vi "Get Array as Variant.vi"(8 "error in (no error)":errorcluster, 10 "Variant (Data Type)":variant, 11 "JSON Value in":refnum<class "JSON Value.lvclass">) -> (0 "error out":errorcluster, 2 "Default VData":variant)   [LabVIEW 2011, in "Variant JSON.lvlib"]
uses:
  Variant JSON.lvlib
  JSON Value/JSON Value.lvclass
  JSON Scalar/Get as I32.vi
  JSON Scalar/Get as I64.vi
  JSON Scalar/Get as U32.vi
  JSON Scalar/Get as SGL.vi
  JSON Scalar/Get as DBL.vi
  JSON Scalar/Get as EXT.vi
  JSON Scalar/Get as Boolean.vi
  JSON Scalar/Get as Text.vi
  JSON Scalar/Get as Path.vi
  JSON Value/Get as Waveform.vi
  JSON Scalar/Get as Timestamp.vi
  JSON Scalar/Get as U64.vi
  <vilib>/Utility/VariantDataType/VariantType.lvlib
  Get Polymorphic/JSON GetSet.lvlib
  JSON Scalar/JSON Scalar.lvclass
  JSON Object/JSON Object.lvclass
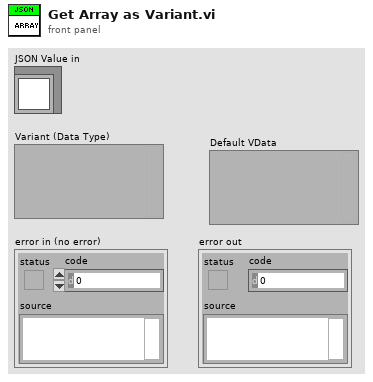
[diagram p1: front panel]
types:
  T1 = typedef "VariantType.lvlib/Type.ctl" = enum8{"Invalid Type", "Void", "I8", "I16", "I32", "I64", "U8", "U16", "U32", "U64", "Single Float", "Double Float", "Extended Float", "Single Complex", "Double Complex", "Extended Complex", "Enum U8", "Enum U16", "Enum U32", "Enum U64", "Single Float With Unit", "Double Float With Unit", "Extended Float With Unit", "Single Complex with Unit", "Double Complex with Unit", "Extended Complex with Unit", "Boolean", "String", "Path", "Picture", "Tag", "Array", "Cluster", "Variant", "LV Variant", "Waveform", "Timestamp", "Digital Waveform", "Digital Data", "ExpressData", "Refnum", "External Data", "VI", "Poly VI", "LabVIEW Class Instance", "Fixed Point"}
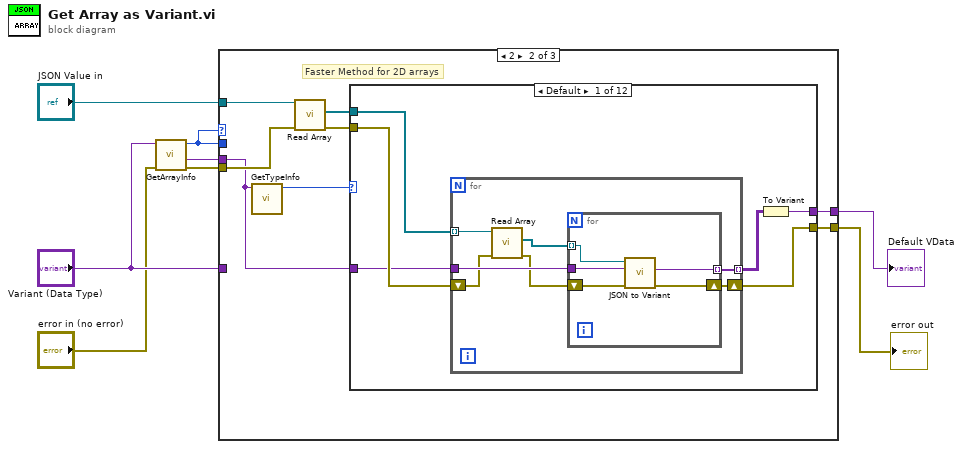
[diagram p0: block diagram]
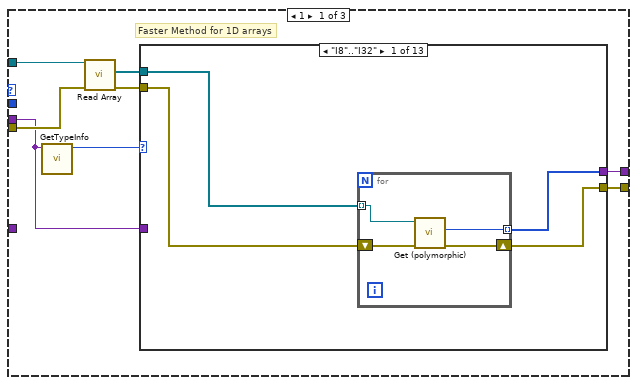
[diagram p2: hidden frame]
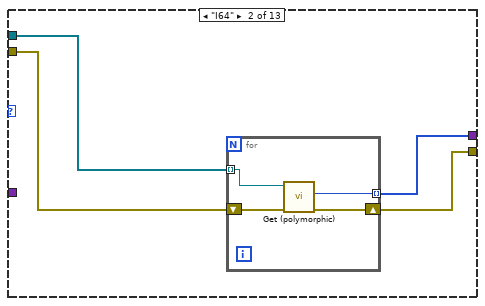
[diagram p3: hidden frame]
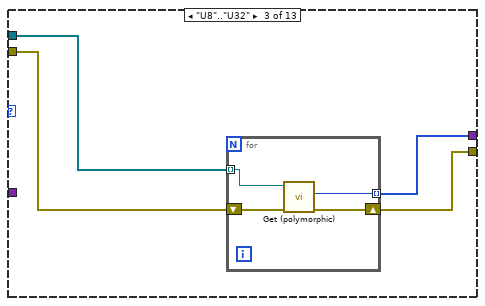
[diagram p4: hidden frame]
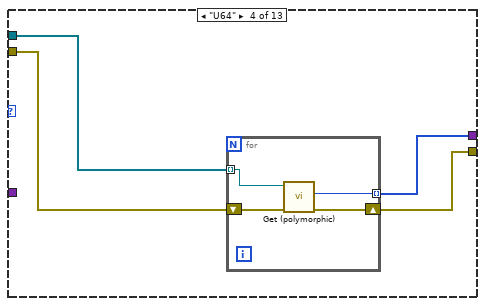
[diagram p5: hidden frame]
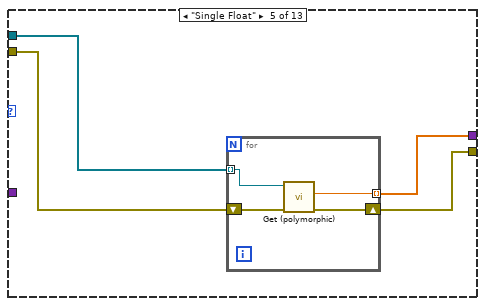
[diagram p6: hidden frame]
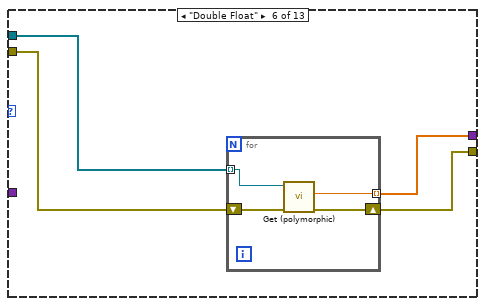
[diagram p7: hidden frame]
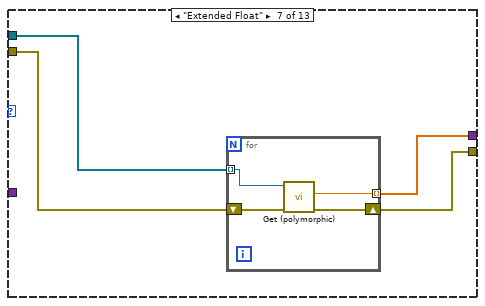
[diagram p8: hidden frame]
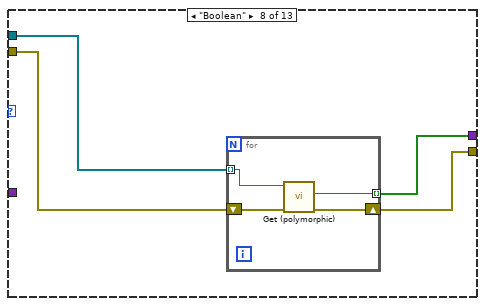
[diagram p9: hidden frame]
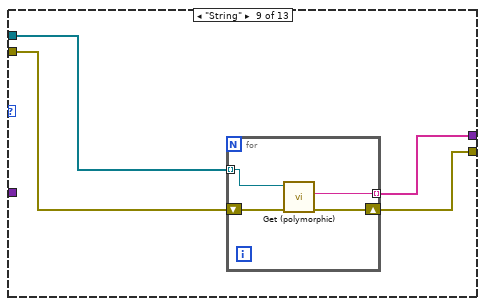
[diagram p10: hidden frame]
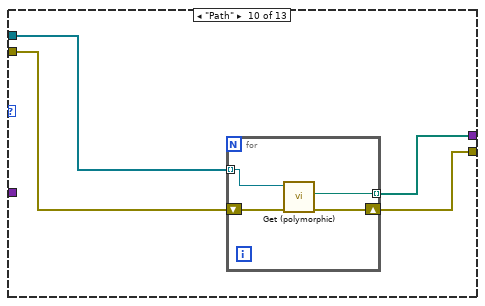
[diagram p11: hidden frame]
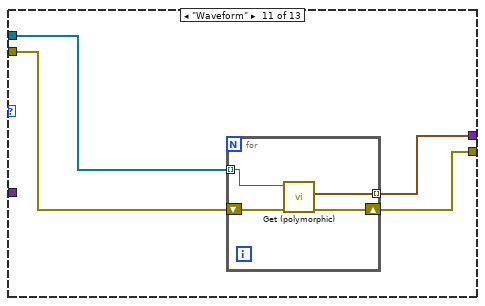
[diagram p12: hidden frame]
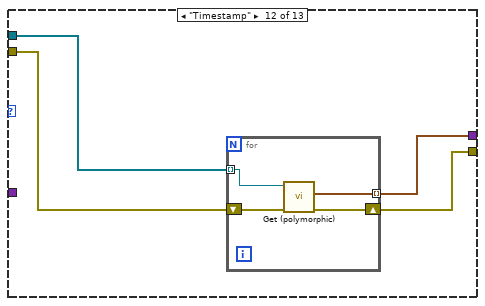
[diagram p13: hidden frame]
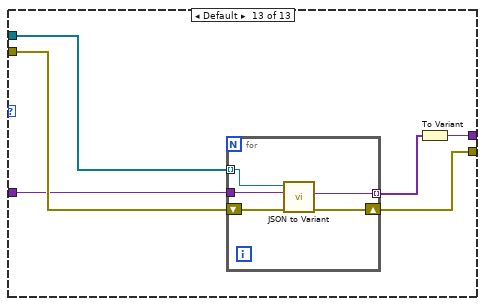
[diagram p14: hidden frame]
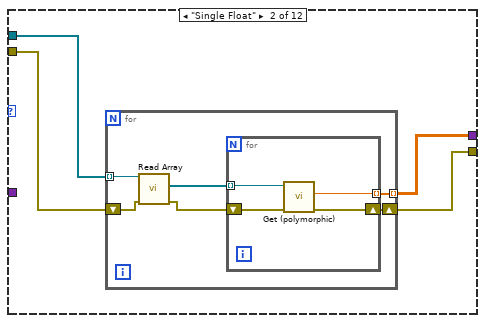
[diagram p15: hidden frame]
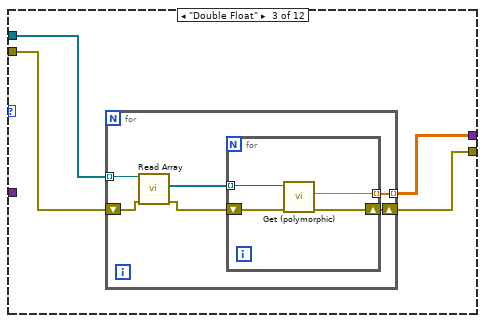
[diagram p16: hidden frame]
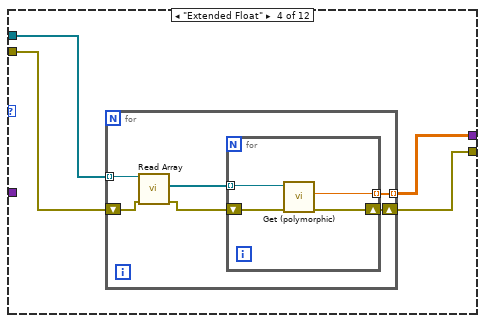
[diagram p17: hidden frame]
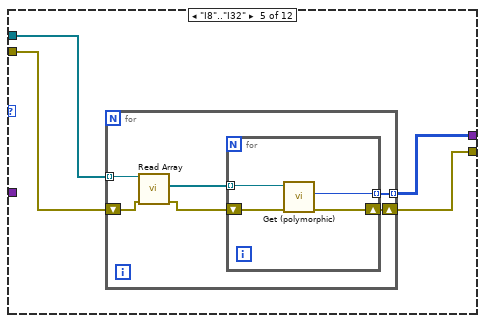
[diagram p18: hidden frame]
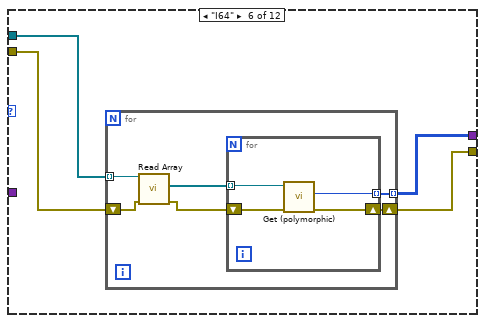
[diagram p19: hidden frame]
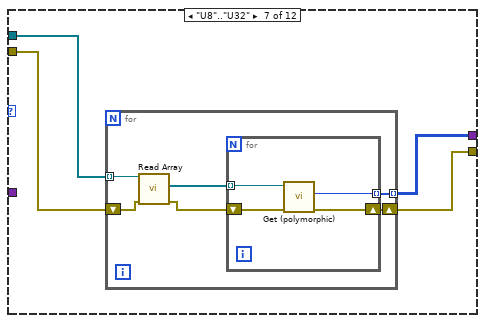
[diagram p20: hidden frame]
diagram:
  n1 = call <vilib>:"GetArrayInfo.vi"("error in (no error)"="error in (no error)", "Variant"="Variant (Data Type)") -> ("error out"=w4:errorcluster, "ArrayElement"=w8:variant, "NDims"=w1:i32)  [unwired: 6 in, 1 out]
  n2 = case shown="2" w1 {
    tunnel: w8 -> [w10 w125 w315]
    tunnel: "Variant (Data Type)" -> [_ _ w314]
    tunnel: [w14 w129 w310] -> w6
    tunnel: [w11 w126 w307] -> w5
    tunnel: w1 -> [_ _ w306]
    tunnel: w4 -> [w13 w128 w305]
    tunnel: "JSON Value in" -> [w16 w131 w304]
    frame 1 {
      # "Faster Method for 1D arrays"
      n3 = call <vilib>:"GetTypeInfo.vi"("Variant"=w10) -> ("Type Enum"=w9:T1)  [unwired: 6 in, 4 out]
      n4 = call-dynamic "Read Array.vi"("error in (no error)"=w13, "JSON Value In"=w16) -> ("error out"=w12:errorcluster, "Array"=w15:refnum<class "JSON Value.lvclass">[])  [unwired: 7 in, 1 out]
      n5 = case shown="\"I8\"..\"I32\"" w9 {
        tunnel: w15 -> [w20 w28 w36 w44 w52 w60 w68 w76 w84 w92 w100 w108 w118]
        tunnel: [w19 w27 w35 w43 w51 w59 w67 w75 w83 w91 w99 w107 w113] -> w14
        tunnel: w12 -> [w17 w25 w33 w41 w49 w57 w65 w73 w81 w89 w97 w105 w116]
        tunnel: [w18 w26 w34 w42 w50 w58 w66 w74 w82 w90 w98 w106 w115] -> w11
        tunnel: w10 -> [_ _ _ _ _ _ _ _ _ _ _ _ w114]
        frame "I8".."I32" {
          n6 = for {
            tunnel: w20 -> [w24] mode=indexing
            tunnel: [w23] -> w19 mode=indexing
            shift-right: [w21] -> w18
            shift-left: w17 -> [w22]
            n7 = call-poly "Get (polymorphic).vi"("error in (no error)"=w22, "JSON Scalar in"=w24) -> ("error out"=w21:errorcluster, "Number"=w23:i32)  [unwired: 7 in, 1 out]
          }
        }
        frame "I64" {
          n8 = for {
            tunnel: w28 -> [w32] mode=indexing
            tunnel: [w31] -> w27 mode=indexing
            shift-right: [w29] -> w26
            shift-left: w25 -> [w30]
            n9 = call-poly "Get (polymorphic).vi"("error in (no error)"=w30, "JSON Scalar in"=w32) -> ("error out"=w29:errorcluster, "Number"=w31:i64)  [unwired: 7 in, 1 out]
          }
        }
        frame "U8".."U32" {
          n10 = for {
            tunnel: w36 -> [w40] mode=indexing
            tunnel: [w39] -> w35 mode=indexing
            shift-right: [w37] -> w34
            shift-left: w33 -> [w38]
            n11 = call-poly "Get (polymorphic).vi"("error in (no error)"=w38, "JSON Scalar in"=w40) -> ("error out"=w37:errorcluster, "Number"=w39:u32)  [unwired: 7 in, 1 out]
          }
        }
        frame "U64" {
          n12 = for {
            tunnel: w44 -> [w48] mode=indexing
            tunnel: [w47] -> w43 mode=indexing
            shift-right: [w45] -> w42
            shift-left: w41 -> [w46]
            n13 = call-poly "Get (polymorphic).vi"("error in (no error)"=w46, "JSON Scalar in"=w48) -> ("error out"=w45:errorcluster, "Number"=w47:i64)  [unwired: 7 in, 1 out]
          }
        }
        frame "Single Float" {
          n14 = for {
            tunnel: w52 -> [w56] mode=indexing
            tunnel: [w55] -> w51 mode=indexing
            shift-right: [w53] -> w50
            shift-left: w49 -> [w54]
            n15 = call-poly "Get (polymorphic).vi"("error in (no error)"=w54, "JSON Value in"=w56) -> ("error out"=w53:errorcluster, "Number"=w55:sgl)  [unwired: 7 in, 1 out]
          }
        }
        frame "Double Float" {
          n16 = for {
            tunnel: w60 -> [w64] mode=indexing
            tunnel: [w63] -> w59 mode=indexing
            shift-right: [w61] -> w58
            shift-left: w57 -> [w62]
            n17 = call-poly "Get (polymorphic).vi"("error in (no error)"=w62, "JSON Value in"=w64) -> ("error out"=w61:errorcluster, "Number"=w63:dbl)  [unwired: 7 in, 1 out]
          }
        }
        frame "Extended Float" {
          n18 = for {
            tunnel: w68 -> [w72] mode=indexing
            tunnel: [w71] -> w67 mode=indexing
            shift-right: [w69] -> w66
            shift-left: w65 -> [w70]
            n19 = call-poly "Get (polymorphic).vi"("error in (no error)"=w70, "JSON Value in"=w72) -> ("error out"=w69:errorcluster, "Number"=w71:ext)  [unwired: 7 in, 1 out]
          }
        }
        frame "Boolean" {
          n20 = for {
            tunnel: w76 -> [w80] mode=indexing
            tunnel: [w79] -> w75 mode=indexing
            shift-right: [w77] -> w74
            shift-left: w73 -> [w78]
            n21 = call-poly "Get (polymorphic).vi"("error in (no error)"=w78, "JSON Value in"=w80) -> ("error out"=w77:errorcluster, "Boolean"=w79:bool)  [unwired: 7 in, 1 out]
          }
        }
        frame "String" {
          n22 = for {
            tunnel: w84 -> [w88] mode=indexing
            tunnel: [w87] -> w83 mode=indexing
            shift-right: [w85] -> w82
            shift-left: w81 -> [w86]
            n23 = call-poly "Get (polymorphic).vi"("error in (no error)"=w86, "JSON Scalar in"=w88) -> ("error out"=w85:errorcluster, "LabVIEW Text"=w87:string)  [unwired: 7 in, 1 out]
          }
        }
        frame "Path" {
          n24 = for {
            tunnel: w92 -> [w96] mode=indexing
            tunnel: [w95] -> w91 mode=indexing
            shift-right: [w93] -> w90
            shift-left: w89 -> [w94]
            n25 = call-poly "Get (polymorphic).vi"("error in (no error)"=w94, "JSON Scalar in"=w96) -> ("error out"=w93:errorcluster, "path"=w95:path)  [unwired: 7 in, 1 out]
          }
        }
        frame "Waveform" {
          n26 = for {
            tunnel: w100 -> [w104] mode=indexing
            tunnel: [w103] -> w99 mode=indexing
            shift-right: [w101] -> w98
            shift-left: w97 -> [w102]
            n27 = call-poly "Get (polymorphic).vi"("error in (no error)"=w102, "JSON Value In"=w104) -> ("error out"=w101:errorcluster, "Waveform"=w103:waveform(dbl))  [unwired: 7 in, 1 out]
          }
        }
        frame "Timestamp" {
          n28 = for {
            tunnel: w108 -> [w112] mode=indexing
            tunnel: [w111] -> w107 mode=indexing
            shift-right: [w109] -> w106
            shift-left: w105 -> [w110]
            n29 = call-poly "Get (polymorphic).vi"("error in (no error)"=w110, "JSON Value in"=w112) -> ("error out"=w109:errorcluster, "Time Stamp"=w111:timestamp)  [unwired: 7 in, 1 out]
          }
        }
        frame Default {
          n30 = for {
            tunnel: w114 -> [w123]
            tunnel: w118 -> [w122] mode=indexing
            tunnel: [w121] -> w117 mode=indexing
            shift-right: [w119] -> w115
            shift-left: w116 -> [w120]
            n31 = call "JSON to Variant.vi"("error in (no error)"=w120, "Variant (Data Type)"=w123, "JSON Value"=w122) -> ("error out"=w119:errorcluster, "Variant out"=w121:variant)  [unwired: 7 in]
          }
          n32 = To Variant(anything=w117) -> (Variant=w113:variant)
        }
      }
    }
    frame 2 {
      # "Faster Method for 2D arrays"
      n33 = call <vilib>:"GetTypeInfo.vi"("Variant"=w125) -> ("Type Enum"=w124:T1)  [unwired: 6 in, 4 out]
      n34 = call-dynamic "Read Array.vi"("error in (no error)"=w128, "JSON Value In"=w131) -> ("error out"=w127:errorcluster, "Array"=w130:refnum<class "JSON Value.lvclass">[])  [unwired: 7 in, 1 out]
      n35 = case shown="Default" w124 {
        tunnel: w130 -> [w132 w153 w167 w181 w195 w209 w223 w237 w251 w265 w279 w293]
        tunnel: [w133 w152 w166 w180 w194 w208 w222 w236 w250 w264 w278 w292] -> w129
        tunnel: w127 -> [w136 w150 w164 w178 w192 w206 w220 w234 w248 w262 w276 w290]
        tunnel: [w135 w151 w165 w179 w193 w207 w221 w235 w249 w263 w277 w291] -> w126
        tunnel: w125 -> [w134 _ _ _ _ _ _ _ _ _ _ _]
        frame Default {
          n36 = for {
            tunnel: [w144] -> w137 mode=indexing
            tunnel: w134 -> [w142]
            tunnel: w132 -> [w141] mode=indexing
            shift-right: [w143] -> w135
            shift-left: w136 -> [w139]
            n37 = call-dynamic "Read Array.vi"("error in (no error)"=w139, "JSON Value In"=w141) -> ("error out"=w138:errorcluster, "Array"=w140:refnum<class "JSON Value.lvclass">[])  [unwired: 7 in, 1 out]
            n38 = for {
              tunnel: w142 -> [w149]
              tunnel: w140 -> [w148] mode=indexing
              tunnel: [w147] -> w144 mode=indexing
              shift-right: [w145] -> w143
              shift-left: w138 -> [w146]
              n39 = call "JSON to Variant.vi"("error in (no error)"=w146, "Variant (Data Type)"=w149, "JSON Value"=w148) -> ("error out"=w145:errorcluster, "Variant out"=w147:variant)  [unwired: 7 in]
            }
          }
          n40 = To Variant(anything=w137) -> (Variant=w133:variant)
        }
        frame "Single Float" {
          n41 = for {
            tunnel: w153 -> [w157] mode=indexing
            tunnel: [w159] -> w152 mode=indexing
            shift-right: [w158] -> w151
            shift-left: w150 -> [w155]
            n42 = call-dynamic "Read Array.vi"("error in (no error)"=w155, "JSON Value In"=w157) -> ("error out"=w154:errorcluster, "Array"=w156:refnum<class "JSON Value.lvclass">[])  [unwired: 7 in, 1 out]
            n43 = for {
              tunnel: w156 -> [w163] mode=indexing
              tunnel: [w162] -> w159 mode=indexing
              shift-right: [w160] -> w158
              shift-left: w154 -> [w161]
              n44 = call-poly "Get (polymorphic).vi"("error in (no error)"=w161, "JSON Value in"=w163) -> ("error out"=w160:errorcluster, "Number"=w162:sgl)  [unwired: 7 in, 1 out]
            }
          }
        }
        frame "Double Float" {
          n45 = for {
            tunnel: w167 -> [w171] mode=indexing
            tunnel: [w173] -> w166 mode=indexing
            shift-right: [w172] -> w165
            shift-left: w164 -> [w169]
            n46 = call-dynamic "Read Array.vi"("error in (no error)"=w169, "JSON Value In"=w171) -> ("error out"=w168:errorcluster, "Array"=w170:refnum<class "JSON Value.lvclass">[])  [unwired: 7 in, 1 out]
            n47 = for {
              tunnel: w170 -> [w177] mode=indexing
              tunnel: [w176] -> w173 mode=indexing
              shift-right: [w174] -> w172
              shift-left: w168 -> [w175]
              n48 = call-poly "Get (polymorphic).vi"("error in (no error)"=w175, "JSON Value in"=w177) -> ("error out"=w174:errorcluster, "Number"=w176:dbl)  [unwired: 7 in, 1 out]
            }
          }
        }
        frame "Extended Float" {
          n49 = for {
            tunnel: w181 -> [w185] mode=indexing
            tunnel: [w187] -> w180 mode=indexing
            shift-right: [w186] -> w179
            shift-left: w178 -> [w183]
            n50 = call-dynamic "Read Array.vi"("error in (no error)"=w183, "JSON Value In"=w185) -> ("error out"=w182:errorcluster, "Array"=w184:refnum<class "JSON Value.lvclass">[])  [unwired: 7 in, 1 out]
            n51 = for {
              tunnel: w184 -> [w191] mode=indexing
              tunnel: [w190] -> w187 mode=indexing
              shift-right: [w188] -> w186
              shift-left: w182 -> [w189]
              n52 = call-poly "Get (polymorphic).vi"("error in (no error)"=w189, "JSON Value in"=w191) -> ("error out"=w188:errorcluster, "Number"=w190:ext)  [unwired: 7 in, 1 out]
            }
          }
        }
        frame "I8".."I32" {
          n53 = for {
            tunnel: w195 -> [w199] mode=indexing
            tunnel: [w201] -> w194 mode=indexing
            shift-right: [w200] -> w193
            shift-left: w192 -> [w197]
            n54 = call-dynamic "Read Array.vi"("error in (no error)"=w197, "JSON Value In"=w199) -> ("error out"=w196:errorcluster, "Array"=w198:refnum<class "JSON Value.lvclass">[])  [unwired: 7 in, 1 out]
            n55 = for {
              tunnel: w198 -> [w205] mode=indexing
              tunnel: [w204] -> w201 mode=indexing
              shift-right: [w202] -> w200
              shift-left: w196 -> [w203]
              n56 = call-poly "Get (polymorphic).vi"("error in (no error)"=w203, "JSON Scalar in"=w205) -> ("error out"=w202:errorcluster, "Number"=w204:i32)  [unwired: 7 in, 1 out]
            }
          }
        }
        frame "I64" {
          n57 = for {
            tunnel: w209 -> [w213] mode=indexing
            tunnel: [w215] -> w208 mode=indexing
            shift-right: [w214] -> w207
            shift-left: w206 -> [w211]
            n58 = call-dynamic "Read Array.vi"("error in (no error)"=w211, "JSON Value In"=w213) -> ("error out"=w210:errorcluster, "Array"=w212:refnum<class "JSON Value.lvclass">[])  [unwired: 7 in, 1 out]
            n59 = for {
              tunnel: w212 -> [w219] mode=indexing
              tunnel: [w218] -> w215 mode=indexing
              shift-right: [w216] -> w214
              shift-left: w210 -> [w217]
              n60 = call-poly "Get (polymorphic).vi"("error in (no error)"=w217, "JSON Scalar in"=w219) -> ("error out"=w216:errorcluster, "Number"=w218:i64)  [unwired: 7 in, 1 out]
            }
          }
        }
        frame "U8".."U32" {
          n61 = for {
            tunnel: w223 -> [w227] mode=indexing
            tunnel: [w229] -> w222 mode=indexing
            shift-right: [w228] -> w221
            shift-left: w220 -> [w225]
            n62 = call-dynamic "Read Array.vi"("error in (no error)"=w225, "JSON Value In"=w227) -> ("error out"=w224:errorcluster, "Array"=w226:refnum<class "JSON Value.lvclass">[])  [unwired: 7 in, 1 out]
            n63 = for {
              tunnel: w226 -> [w233] mode=indexing
              tunnel: [w232] -> w229 mode=indexing
              shift-right: [w230] -> w228
              shift-left: w224 -> [w231]
              n64 = call-poly "Get (polymorphic).vi"("error in (no error)"=w231, "JSON Scalar in"=w233) -> ("error out"=w230:errorcluster, "Number"=w232:u32)  [unwired: 7 in, 1 out]
            }
          }
        }
        frame "U64" {
          n65 = for {
            tunnel: w237 -> [w241] mode=indexing
            tunnel: [w243] -> w236 mode=indexing
            shift-right: [w242] -> w235
            shift-left: w234 -> [w239]
            n66 = call-dynamic "Read Array.vi"("error in (no error)"=w239, "JSON Value In"=w241) -> ("error out"=w238:errorcluster, "Array"=w240:refnum<class "JSON Value.lvclass">[])  [unwired: 7 in, 1 out]
            n67 = for {
              tunnel: w240 -> [w247] mode=indexing
              tunnel: [w246] -> w243 mode=indexing
              shift-right: [w244] -> w242
              shift-left: w238 -> [w245]
              n68 = call-poly "Get (polymorphic).vi"("error in (no error)"=w245, "JSON Scalar in"=w247) -> ("error out"=w244:errorcluster, "Number"=w246:u64)  [unwired: 7 in, 1 out]
            }
          }
        }
        frame "String" {
          n69 = for {
            tunnel: w251 -> [w255] mode=indexing
            tunnel: [w257] -> w250 mode=indexing
            shift-right: [w256] -> w249
            shift-left: w248 -> [w253]
            n70 = call-dynamic "Read Array.vi"("error in (no error)"=w253, "JSON Value In"=w255) -> ("error out"=w252:errorcluster, "Array"=w254:refnum<class "JSON Value.lvclass">[])  [unwired: 7 in, 1 out]
            n71 = for {
              tunnel: w254 -> [w261] mode=indexing
              tunnel: [w260] -> w257 mode=indexing
              shift-right: [w258] -> w256
              shift-left: w252 -> [w259]
              n72 = call-poly "Get (polymorphic).vi"("error in (no error)"=w259, "JSON Scalar in"=w261) -> ("error out"=w258:errorcluster, "LabVIEW Text"=w260:string)  [unwired: 7 in, 1 out]
            }
          }
        }
        frame "Path" {
          n73 = for {
            tunnel: w265 -> [w269] mode=indexing
            tunnel: [w271] -> w264 mode=indexing
            shift-right: [w270] -> w263
            shift-left: w262 -> [w267]
            n74 = call-dynamic "Read Array.vi"("error in (no error)"=w267, "JSON Value In"=w269) -> ("error out"=w266:errorcluster, "Array"=w268:refnum<class "JSON Value.lvclass">[])  [unwired: 7 in, 1 out]
            n75 = for {
              tunnel: w268 -> [w275] mode=indexing
              tunnel: [w274] -> w271 mode=indexing
              shift-right: [w272] -> w270
              shift-left: w266 -> [w273]
              n76 = call-poly "Get (polymorphic).vi"("error in (no error)"=w273, "JSON Scalar in"=w275) -> ("error out"=w272:errorcluster, "path"=w274:path)  [unwired: 7 in, 1 out]
            }
          }
        }
        frame "Timestamp" {
          n77 = for {
            tunnel: w279 -> [w283] mode=indexing
            tunnel: [w285] -> w278 mode=indexing
            shift-right: [w284] -> w277
            shift-left: w276 -> [w281]
            n78 = call-dynamic "Read Array.vi"("error in (no error)"=w281, "JSON Value In"=w283) -> ("error out"=w280:errorcluster, "Array"=w282:refnum<class "JSON Value.lvclass">[])  [unwired: 7 in, 1 out]
            n79 = for {
              tunnel: w282 -> [w289] mode=indexing
              tunnel: [w288] -> w285 mode=indexing
              shift-right: [w286] -> w284
              shift-left: w280 -> [w287]
              n80 = call-poly "Get (polymorphic).vi"("error in (no error)"=w287, "JSON Value in"=w289) -> ("error out"=w286:errorcluster, "Time Stamp"=w288:timestamp)  [unwired: 7 in, 1 out]
            }
          }
        }
        frame "Waveform" {
          n81 = for {
            tunnel: w293 -> [w297] mode=indexing
            tunnel: [w299] -> w292 mode=indexing
            shift-right: [w298] -> w291
            shift-left: w290 -> [w295]
            n82 = call-dynamic "Read Array.vi"("error in (no error)"=w295, "JSON Value In"=w297) -> ("error out"=w294:errorcluster, "Array"=w296:refnum<class "JSON Value.lvclass">[])  [unwired: 7 in, 1 out]
            n83 = for {
              tunnel: w296 -> [w303] mode=indexing
              tunnel: [w302] -> w299 mode=indexing
              shift-right: [w300] -> w298
              shift-left: w294 -> [w301]
              n84 = call-poly "Get (polymorphic).vi"("error in (no error)"=w301, "JSON Value In"=w303) -> ("error out"=w300:errorcluster, "Waveform"=w302:waveform(dbl))  [unwired: 7 in, 1 out]
            }
          }
        }
      }
    }
    frame Default {
      # "General (but slow) method works on any array dimension"
      n85 = call "JSON to MultiD Array.vi"("error in (no error)"=w305, "ArrayElementType"=w315, "NDims"=w306, "JSON Value in"=w304) -> ("error out"=w309:errorcluster, "Dimensions"=w311:i32[], "Array Elements"=w308:variant[])  [unwired: 5 in]
      n86 = Equal To 0?(x=w311) -> (x = 0?=w312:bool[])
      n87 = Or Array Elements "Any zero"(Boolean array=w312) -> (logical OR=w313:bool)
      n88 = case shown="True" w313 {
        tunnel: [w323 w325] -> w307
        tunnel: w308 -> [w322 _]
        tunnel: w315 -> [w321 _]
        tunnel: w309 -> [w320 w327]
        tunnel: [w317 w326] -> w310
        tunnel: w311 -> [w316 _]
        tunnel: w314 -> [_ w324]
        frame False {
          n89 = call <userlib>:"Array of VData to VArray__ogtk.vi"("error in (no error)"=w320, "Element Type (when empty)"=w321, "1D Array of VData"=w322) -> ("error out"=w318:errorcluster, "VArray"=w319:variant)  [unwired: 7 in]
          n90 = call <userlib>:"Reshape 1D Array__ogtk.vi"("error in (no error)"=w318, "Size(s)"=w316, "1D Array"=w319) -> ("error out"=w323:errorcluster, "Reshaped VArray"=w317:variant)  [unwired: 7 in]
        }
        frame True {
          # "Any zero-size dimentions means we must return an\nempty array."
          n91 = call <userlib>:"Get Default Data from Variant__ogtk.vi"("error in (no error)"=w327, "Variant"=w324) -> ("error out"=w325:errorcluster, "Default VData"=w326:variant)  [unwired: 8 in]
        }
      }
    }
  }
  "Default VData" <- w6
  "error out" <- w5
